vi "CreateOccurance.vi"() -> (0 "Occurrence Refnum":refnum<k4>)   [LabVIEW 2012]
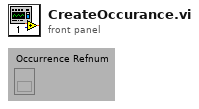
[diagram p1: front panel]
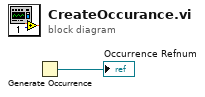
[diagram p0: block diagram]
diagram:
  n1 = Generate Occurrence() -> (→"Occurrence Refnum":refnum<k4>)
